vi "Add Measurement Rows.vi"(8 "error in (no error)":errorcluster, 11 "Measurements in":T1) -> (0 "error out":errorcluster, 3 "Measurements out":T1)   [LabVIEW 2026, in "Settings.lvlib"]
uses:
  controls/UI/Measurement Config.ctl
  controls/UI/Measurement Role.ctl
  Settings.lvlib
  controls/UI/Measurements Config.ctl
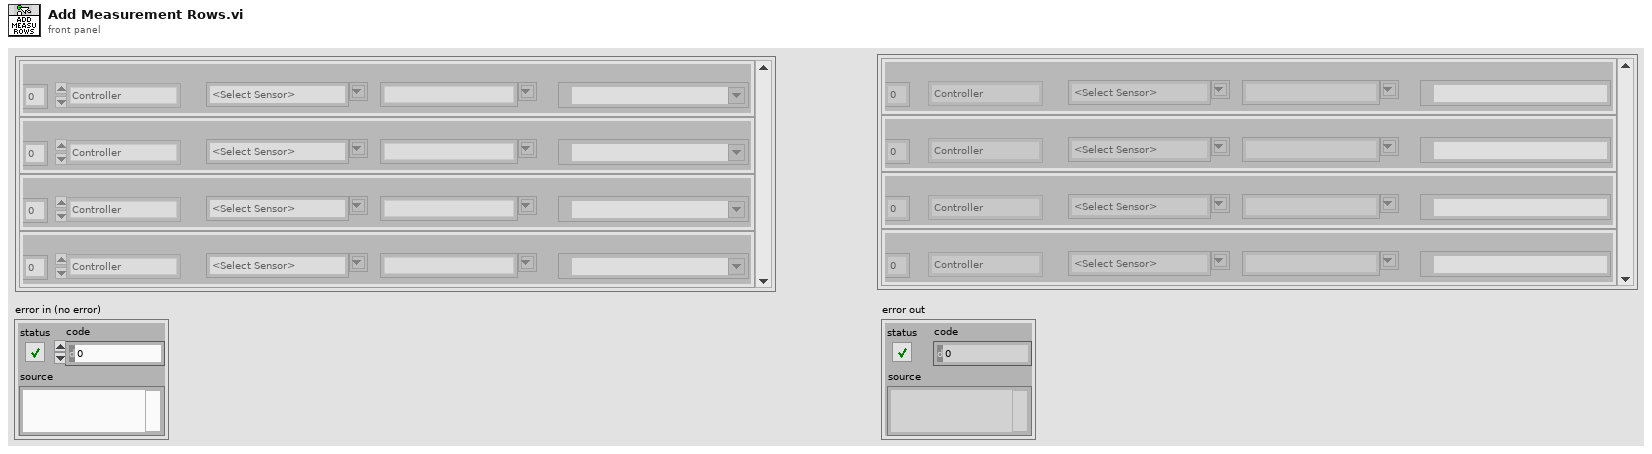
[diagram p1: front panel]
types:
  T1 = typedef "Measurements Config.ctl" = T2[]
  T2 = typedef "Measurement Config.ctl" = cluster{"DAQmx AI Physical Channel":tag, "Serial Numbers":string, "Model Numbers":string, "Role":T3, "Row":i32}
  T3 = typedef "Settings.lvlib/Measurement Role.ctl" = enum16{"Controller", "Reference", "UUT", "Disable", "All"}
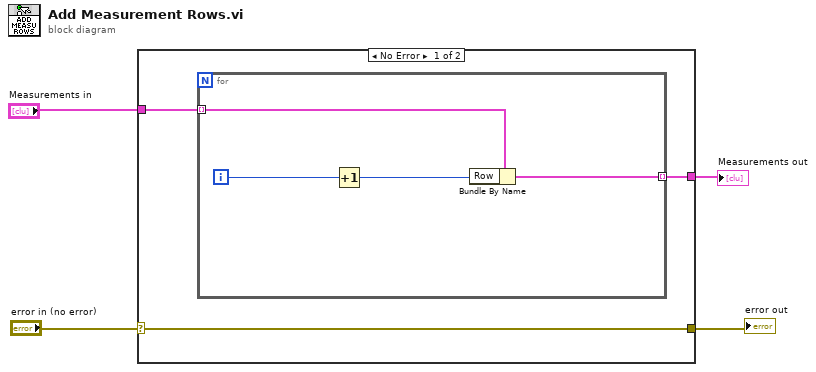
[diagram p0: block diagram]
diagram:
  n1 = case shown="No Error" "error in (no error)" {
    selector: "error in (no error)" -> [w5 w13]
    tunnel: "Measurements in" -> [w7 w12]
    tunnel: [w6 w12] -> w1
    tunnel: [w5 w13] -> w3
    frame No Error {
      n2 = for {
        tunnel: w7 -> [w11] mode=indexing
        tunnel: [w8] -> w6 mode=indexing
        i -> [w10]
        n3 = Increment(x=w10) -> (x+1=w9:i32)
        n4 = Bundle By Name(cluster=w11, "Row"=w9) -> (w8:T2)
      }
    }
    frame Error {
    }
  }
  "error out" <- w3
  "Measurements out" <- w1
